vi "Part 1.vi"(11 "Input":string) -> (3 "Output":i64)   [LabVIEW 2021]
uses:
  <userlib>/_OpenG.lib/array/array.llb/Search 1D Array (I64)__ogtk.vi
panel:
  out "Grid":i64[][](array[numeric])
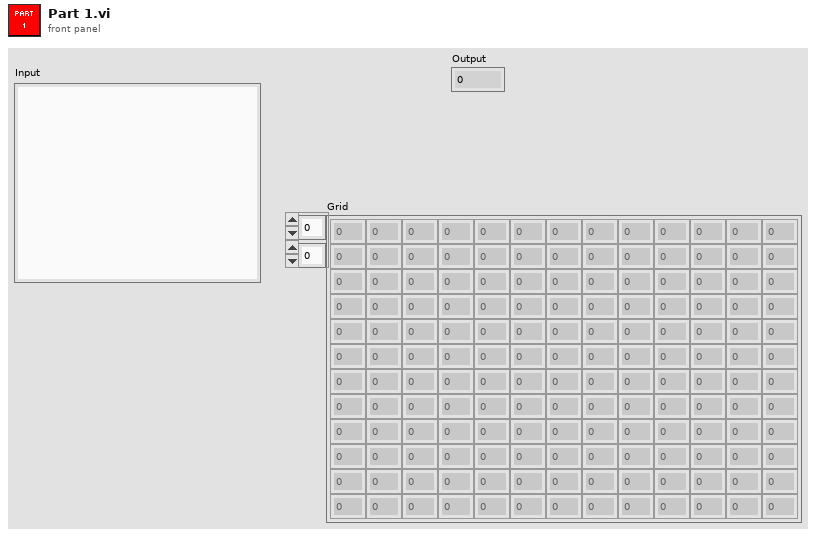
[diagram p1: front panel]
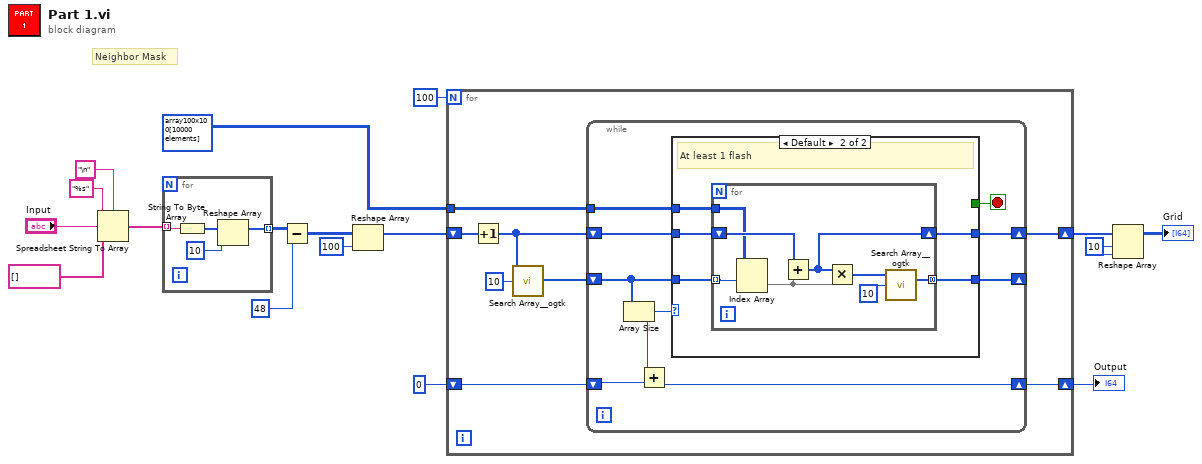
[diagram p0: block diagram]
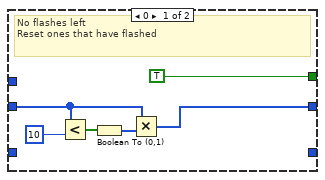
[diagram p2: hidden frame]
diagram:
  w2 = 10 ("dimension size")
  # "Neighbor Mask"
  n1 = Spreadsheet String To Array(delimiter (Tab)="\n", format string="%s", spreadsheet string="Input", array type (2D Dbl)=string[] []) -> (array=w13:string[])
  n2 = for {
    tunnel: w13 -> [w21] mode=indexing
    tunnel: [w19] -> w12 mode=indexing
    n3 = String To Byte Array(string=w21) -> (unsigned byte array=w20:u8[])
    n4 = Reshape Array(w20, 10 ("dimension size")) -> (w19:u8[])
  }
  n5 = Subtract(x=w12, y=i64 48) -> (x-y=w10:i64[][])
  n6 = Reshape Array(w10, 100 ("dimension size")) -> (w5:i64[])
  n7 = for {
    N: 100 -> [_]
    shift-right: [w28] -> w7
    shift-left: w5 -> [w29]
    shift-right: [w26] -> w8
    shift-left: i64 0 -> [w27]
    tunnel: i16[][] array100x100[10000 elements] ("Array") -> [w22]
    n8 = Increment(x=w29) -> (x+1=w25:i64[])
    n9 = call-poly <userlib>:"Search Array__ogtk.vi"("Array"=w25, "Element Data"=i64 10) -> ("Indices of Elements"=w23:i32[])  [unwired: 7 in]
    n10 = while {
      shift-right: [w38] -> w28
      shift-left: w25 -> [w35]
      shift-right: [w34] -> _
      shift-left: w23 -> [w36]
      shift-right: [w31] -> w26
      shift-left: w27 -> [w33]
      tunnel: w22 -> [w30]
      stop <- w37 stop-if-true
      n11 = Array Size(array=w36) -> (size(s)=w32:i32)
      n12 = Add(x=w32, y=w33) -> (x+y=w31:i64)
      n13 = case shown="Default" w32 {
        tunnel: [w39 w47] -> w38
        tunnel: [TRUE _] -> w37
        tunnel: w36 -> [_ w49]
        tunnel: w35 -> [w40 w48]
        tunnel: [_ w46] -> w34
        tunnel: w30 -> [_ w45]
        frame 0 {
          # "No flashes left\nReset ones that have flashed"
          n14 = Less?(x=w40, y=i64 10) -> (x < y?=w43:bool[])
          n15 = Boolean To (0,1)(Boolean=w43) -> (0, 1=w42:i16[])
          n16 = Multiply(x=w40, y=w42) -> (x*y=w39:i64[])
        }
        frame Default {
          # "At least 1 flash"
          n17 = for {
            tunnel: w49 -> [w55] mode=indexing
            shift-right: [w53] -> w47
            shift-left: w48 -> [w54]
            tunnel: [w57] -> w46 mode=concatenating
            tunnel: w45 -> [w52]
            n18 = Index Array(array=w52, index (row)=w55) -> (element=w51:i16[])  [unwired: 1 in]
            n19 = Add(x=w54, y=w51) -> (x+y=w53:i64[])
            n20 = Multiply(x=w53, y=w51) -> (x*y=w50:i64[])
            n21 = call-poly <userlib>:"Search Array__ogtk.vi"("Array"=w50, "Element Data"=i64 10) -> ("Indices of Elements"=w57:i32[])  [unwired: 7 in]
          }
        }
      }
    }
  }
  "Output" <- w8
  n22 = Reshape Array(w7, w2, w2) -> (→"Grid":i64[][])
